vi "SamplingPeriod.vi"() -> ()   [LabVIEW 2020]
panel:
  in  "Sampling period":u32=100
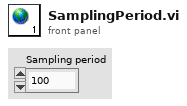
[diagram p1: front panel]
diagram:
